vi "setUp.vi"(8 "error in (no error)":errorcluster, 11 "reference in":refnum<class "Test Notifying Nested Endpoint.lvclass">) -> (0 "error out":errorcluster, 3 "reference out":refnum<class "Test Notifying Nested Endpoint.lvclass">)   [LabVIEW 2020, in "Test Notifying Nested Endpoint.lvclass"]
doc: "setUp runs prior to the test method during test execution. Use this method to initialize any object data required by your tests."
uses:
  Test Notifying Nested Endpoint.lvclass
  <vilib>/addons/_JKI Toolkits/VI Tester/TestCase.llb/TestCase.lvclass
  <vilib>/ActorFramework/Actor/Actor.lvclass
  <vilib>/ActorFramework/Message Queue/Message Queue.lvclass
  Source/Network Endpoint/Network Endpoint/Network Endpoint.lvclass
  Test Harness/AF Queue Stream/AF Queue Stream.lvclass
  Source/Notifying Nested Endpoint/Notifying Nested Endpoint.lvclass
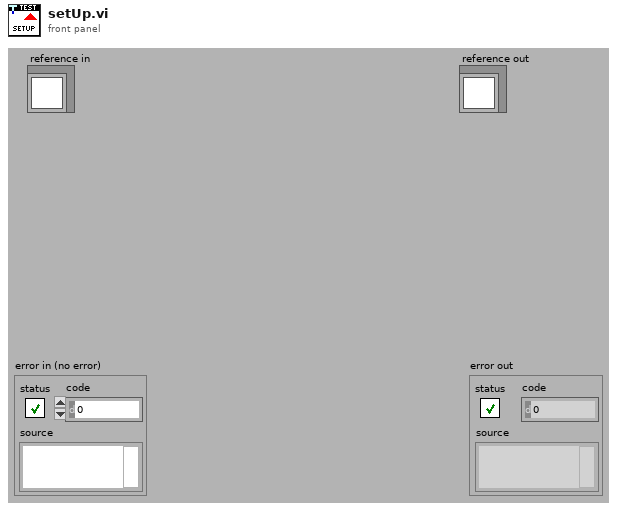
[diagram p1: front panel]
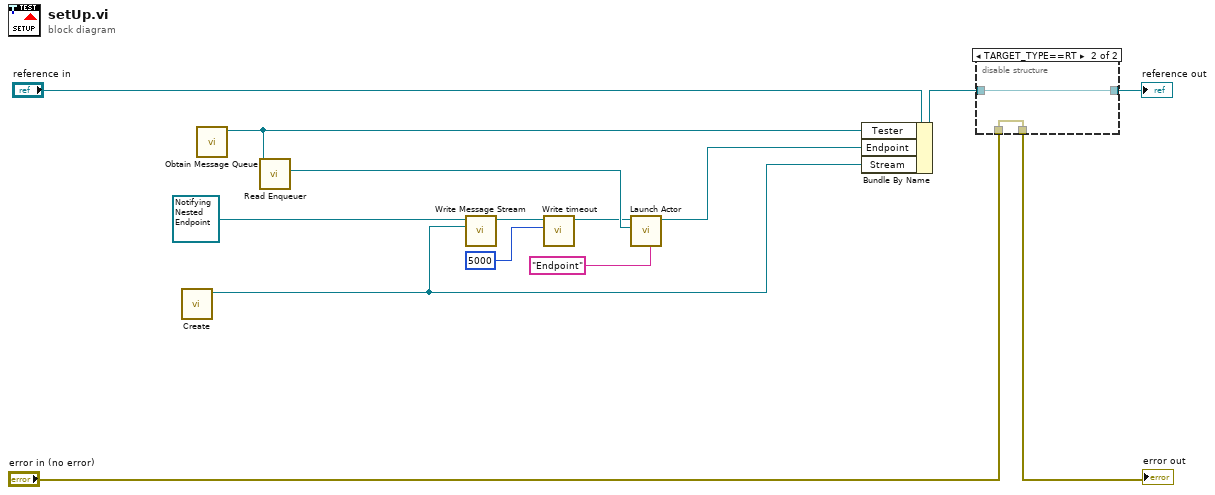
[diagram p0: block diagram]
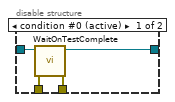
[diagram p2: hidden frame]
diagram:
  n1 = call "Create.vi"() -> ("AF Queue Stream out"=w3:refnum<class "AF Queue Stream.lvclass">)  [unwired: 11 in]
  n2 = call <vilib>:"Obtain Message Queue.vi"() -> ("Message Queue"=w7:refnum<class "Message Queue.lvclass">)  [unwired: 10 in, 1 out]
  n3 = call <vilib>:"Read Enqueuer.vi"("Message Queue"=w7) -> ("Message Enqueuer"=w10:refnum<class "Message Enqueuer.lvclass">)  [unwired: 10 in]
  n4 = call "Write Message Stream.vi"("Message Stream"=w3, "Network Endpoint in"=refnum<class "Notifying Nested Endpoint.lvclass"> refnum ("Notifying Nested Endpoint.lvclass")) -> ("Network Endpoint out"=w6:refnum<class "Notifying Nested Endpoint.lvclass">)  [unwired: 9 in]
  n5 = call "Write timeout.vi"("timeout"=5000, "Network Endpoint in"=w6) -> ("Network Endpoint out"=w5:refnum<class "Notifying Nested Endpoint.lvclass">)  [unwired: 9 in]
  n6 = call <vilib>:"Launch Actor.vi"("Debug Alias"="Endpoint", "Actor-to-Caller Enqueuer"=w10, "Actor"=w5) -> ("Caller-To-Actor Enqueuer"=w8:refnum<class "Message Enqueuer.lvclass">)  [unwired: 7 in, 1 out]
  n7 = Bundle By Name(cluster="reference in", "Tester"=w7, "Endpoint"=w8, "Stream"=w3) -> (w11:refnum<class "Test Notifying Nested Endpoint.lvclass">)
  n8 = disable-structure shown="TARGET_TYPE==RT" {
    disable-tunnel: "error in (no error)" -> [w18 w19]
    disable-tunnel: [w17 w19] -> w14
    disable-tunnel: [w16 w20] -> w12
    disable-tunnel: w11 -> [w15 w20]
    frame condition #0 (active) {
      n9 = call <vilib>:"WaitOnTestComplete.vi"("error in (no error)"=w18, "TestCase in"=w15) -> ("error out"=w17:errorcluster, "TestCase out"=w16:refnum<class "Test Notifying Nested Endpoint.lvclass">)  [unwired: 8 in]
    }
    frame condition #1 {
    }
  }
  "error out" <- w14
  "reference out" <- w12
